vi "Files in a folder to drop down menu.vi"(0 "Ring":u16(ring) items=["hosts.txt", "kabali.txt", "Shortest Path Algorithm.txt", "To Download.txt", "Vijay Saayi voter card reference number.txt"], 2 "OK Button":bool) -> (1 "Path":path, 3 "filenames":string[](array[string]))   [LabVIEW 2014]
panel:
  out "element":string
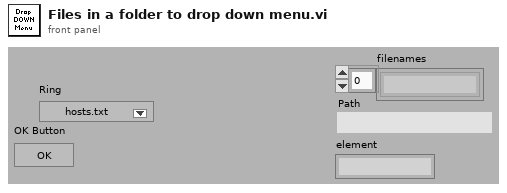
[diagram p1: front panel]
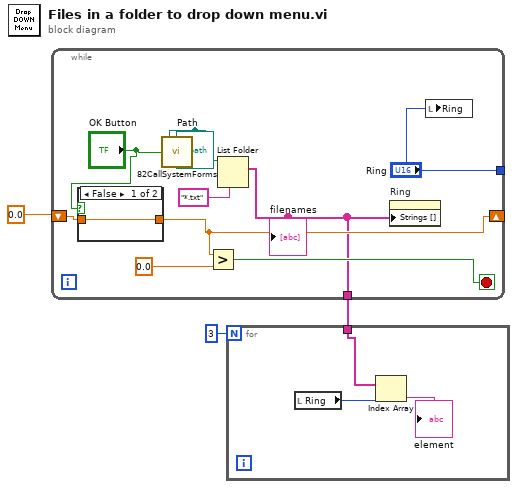
[diagram p0: block diagram]
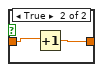
[diagram p2: hidden frame]
diagram:
  n1 = while {
    shift-right: [w6] -> _
    shift-left: 0.0 ("Numeric") -> [w7]
    tunnel: ["Ring"] -> _
    tunnel: [w5] -> w2
    stop <- w9 stop-if-true
    n2 = case shown="False" "OK Button" {
      tunnel: w7 -> [w13 w15]
      tunnel: [w13 w14] -> w6
      frame False {
      }
      frame True {
        n3 = Increment(x=w15) -> (x+1=w14:dbl)
      }
    }
    n4 = call "82CallSystemForms.vi"("OK Button"="OK Button") -> ("Path"=w11:path)  [unwired: 1 in, 2 out]
    "Path" <- w11
    n5 = Greater?(x=w6, y=0.0 ("Numeric")) -> (0:w9:bool)
    n6 = List Folder(path=w11, pattern="*.txt") -> (filenames=w5:string[])  [unwired: 2 in, 3 out]
    "filenames" <- w5
    n7 = property on="Ring" class="Ring (strict)"("Strings []"=w5) -> ()  [unwired: 2 in, 2 out]
    n8 = local write "Ring"("Ring") -> ()
  }
  n9 = for {
    N: 3 -> [_]
    tunnel: w2 -> [w18]
    n10 = local read "Ring"() -> (w17:u16)
    n11 = Index Array(array=w18, index=w17) -> (element=→"element":string)
  }
